vi "Get capillary hexapod fit for move along laser line.vi"() -> ()   [LabVIEW 2013]
uses:
  General GUIs/General-Controler/scan parameters.ctl
  <vilib>/Analysis/NI_AALPro.lvlib
panel:
  in  "Cluster":T2={"Scan parameters"={"Scan Start"=-6.0, "Scan End"=6.0, "Scan Step Size"=3.0, "# Shots Each Step"=3, "single direction?"=TRUE}, "device and variable preamble"="Device = \"PL1-Hexapod,PL1-Hexapod,PL1-Hexapod\"\nVariable = \"xpos,ypos,zpos\""} {"Scan parameters"."Scan Start" format="%#.9p"; "Scan parameters"."Scan End" format="%#.9p"; "Scan parameters"."Scan Step Size" format="%#.9p"}
  out "P(x)":dbl[][](array[numeric])=[[-1.5943478260869566, 0.0013636363636363653], [0.8795652173913043, -0.0009090909090909098]] caption="P(x) ascending order of power." min=0.0 max=127.0 format="%#.6f"
  in  "z values":dbl[](array[numeric])=[0.89, 0.85]
  in  "y values":dbl[](array[numeric])=[-1.61, -1.55]
  in  "x values":dbl[](array[numeric])=[0.0, 22.0]
  out "intercept for HexY":dbl=-1.5943478260869566
  out "slope for Hexy":dbl=0.0013636363636363653
  out "slope for HexZ":dbl=-0.0009090909090909098
  out "intercept for HexZ":dbl=0.8795652173913043
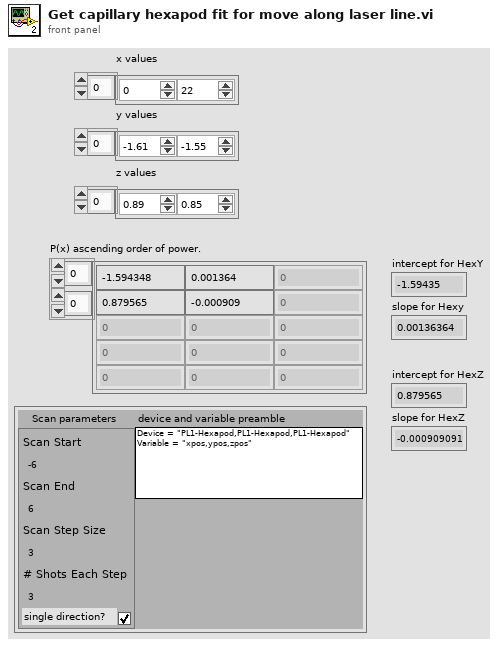
[diagram p1: front panel]
types:
  T1 = typedef "scan parameters.ctl" = cluster{"Scan Start":dbl, "Scan End":dbl, "Scan Step Size":dbl, "# Shots Each Step":u32, "single direction?":bool}
  T2 = cluster{"Scan parameters":T1, "device and variable preamble":string}
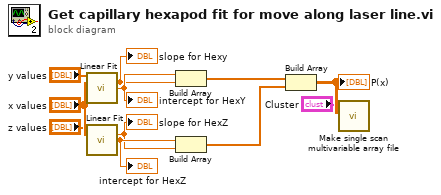
[diagram p0: block diagram]
diagram:
  n1 = call <vilib>:"Linear Fit.vi"("Y"="y values", "X"="x values") -> ("slope"=w10:dbl, "intercept"=w11:dbl)  [unwired: 9 in, 3 out]
  "intercept for HexY" <- w11
  "slope for Hexy" <- w10
  n2 = call <vilib>:"Linear Fit.vi"("Y"="z values", "X"="x values") -> ("slope"=w8:dbl, "intercept"=w9:dbl)  [unwired: 9 in, 3 out]
  "intercept for HexZ" <- w9
  "slope for HexZ" <- w8
  n3 = Build Array(w11, w10) -> (w7:dbl[])
  n4 = Build Array(w9, w8) -> (w6:dbl[])
  n5 = Build Array(w7, w6) -> (w5:dbl[][])
  "P(x)" <- w5
  n6 = call "Make single scan multivariable array file.vi"("P(x)"=w5, "Cluster"="Cluster") -> ()  [unwired: 10 in]
